vi "frw_csv_ini.vi"(8 "error in":errorcluster, 9 "eeg_device":T1, 10 "file_name":string, 11 "folder":path) -> (0 "error out":errorcluster, 3 "path out":path)   [LabVIEW 2013]
uses:
  gui/type_def/device.ctl
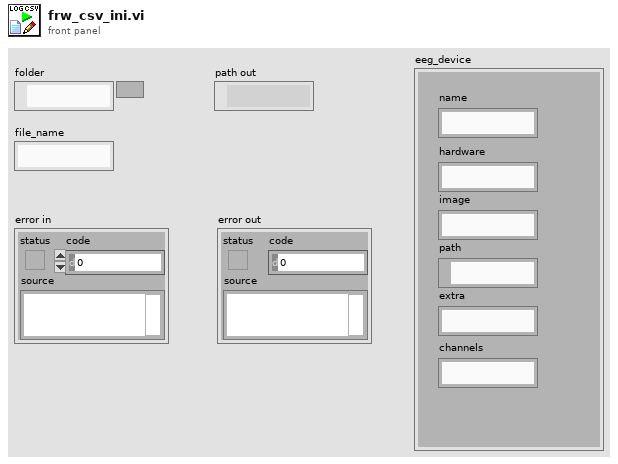
[diagram p1: front panel]
types:
  T1 = typedef "device.ctl" = cluster{"name":string, "hardware":string, "image":string, "path":path, "extra":string, "channels":string}
  T2 = enum16{"open", "replace", "create", "open or create", "replace or create", "replace or create with confirmation"}
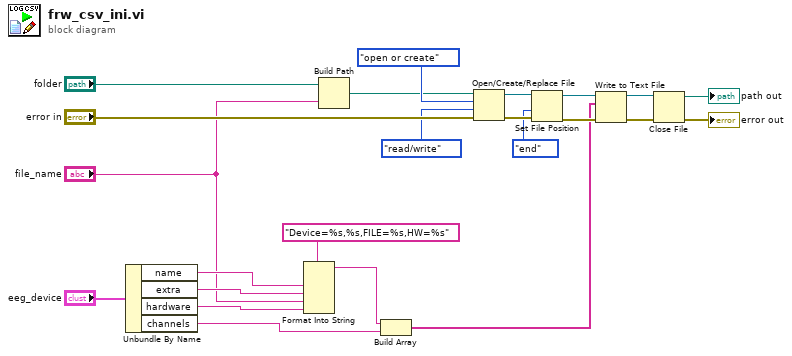
[diagram p0: block diagram]
diagram:
  n1 = Unbundle By Name("eeg_device") -> ("name"=w9:string, "extra"=w8:string, "hardware"=w7:string, "channels"=w5:string)
  n2 = Format Into String(format string="Device=%s,%s,FILE=%s,HW=%s", w9, w8, "file_name", w7) -> (resulting string=w6:string)  [unwired: 2 in, 1 out]
  n3 = Build Path(base path="folder", name or relative path="file_name") -> (appended path=w2:path)
  n4 = Build Array(w6, w5) -> (w4:string[])
  n5 = Open/Create/Replace File(file path (use dialog)=w2, error in="error in", operation (0:open)=T2."open or create", access (0:read/write)=enum16{"read/write", "read-only", "write-only"}."read/write") -> (refnum out=w19:refnum<file>, error out=w21:errorcluster)  [unwired: 3 out]
  n6 = Set File Position(refnum=w19, from (0:start)=enum16{"start", "end", "current"}."end", error in=w21) -> (refnum out=w18:refnum<file>, error out=w17:errorcluster)  [unwired: 1 in]
  n7 = Write to Text File(file (use dialog)=w18, text=w4, error in=w17) -> (refnum out=w15:refnum<file>, error out=w16:errorcluster)  [unwired: 2 out]
  n8 = Close File(refnum=w15, error in=w16) -> (path=→"path out":path, error out=→"error out":errorcluster)
